vi "SetSoftwareLimits.vi"(8 "error in (no error)":errorcluster, 9 "Positive limit (right)":dbl, 10 "Negative limit (left)":dbl, 11 "VISA resource name":refnum<visa-resource-name>) -> (0 "error out":errorcluster)   [LabVIEW 2013]
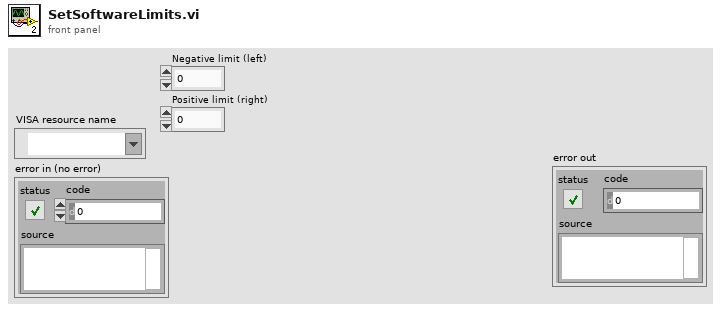
[diagram p1: front panel]
types:
  T1 = cluster{"VISA resource name":refnum<visa-resource-name>, "Device name":string, "Controller address":i32, "error":errorcluster}
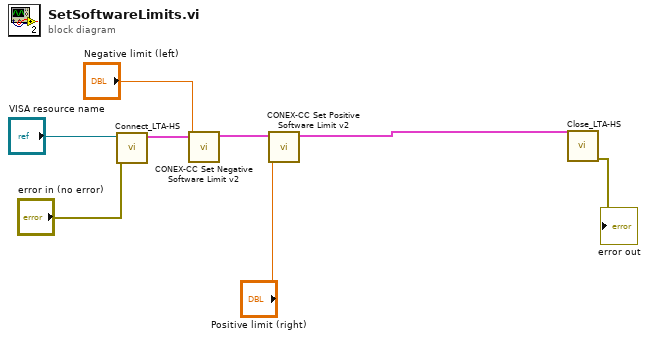
[diagram p0: block diagram]
diagram:
  n1 = call "Connect_LTA-HS.vi"("error in (no error)"="error in (no error)", "VISA resource name"="VISA resource name") -> ("Device Connection Cluster"=w3:T1)  [unwired: 8 in, 1 out]
  n2 = call "CONEX-CC Set Negative Software Limit v2.vi"("Negative limit (left)"="Negative limit (left)", "Connection Cluster in"=w3) -> ("Connection Cluster out"=w2:T1)  [unwired: 9 in]
  n3 = call "CONEX-CC Set Positive Software Limit v2.vi"("Positive limit (right)"="Positive limit (right)", "Connection Cluster in"=w2) -> ("Connection Cluster out"=w1:T1)  [unwired: 9 in]
  n4 = call "Close_LTA-HS.vi"("Connection Cluster in"=w1) -> ("error out"=→"error out":errorcluster)  [unwired: 10 in]
